vi "Local Variables.vi"() -> ()   [LabVIEW 2016]
panel:
  out "Stop":bool
  out "Boolean 3":bool
  out "Boolean 2":bool
  out "Boolean":bool
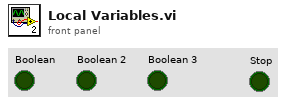
[diagram p1: front panel]
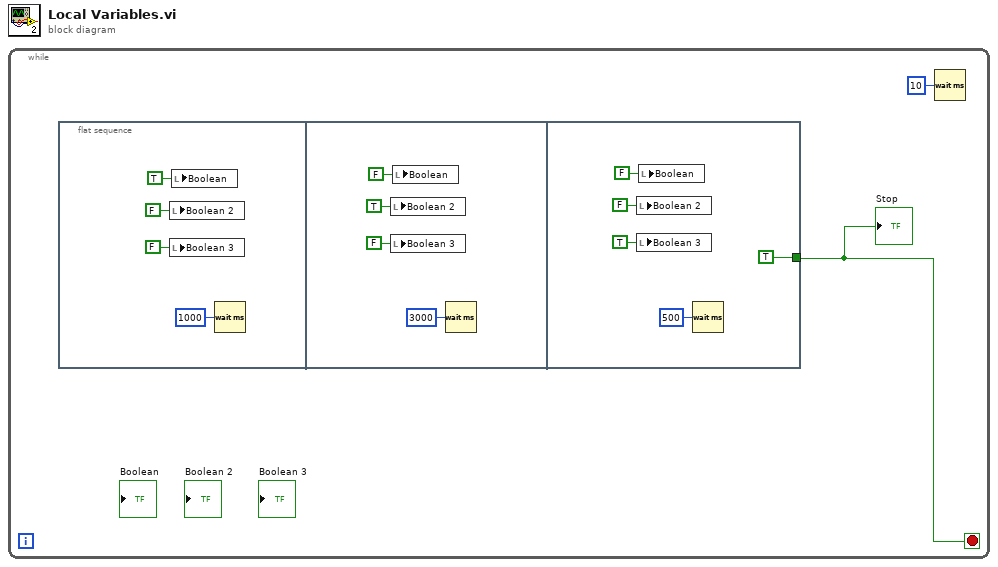
[diagram p0: block diagram]
diagram:
  n1 = while {
    stop <- w2 stop-if-true
    n2 = flat-sequence {
      tunnel: [TRUE] -> w2
      frame #0 {
        n3 = local write "Boolean 2"(FALSE ("Boolean 2")) -> ()
        n4 = local write "Boolean 3"(FALSE ("Boolean 3")) -> ()
        n5 = local write "Boolean"(TRUE ("Boolean")) -> ()
        n6 = Wait (ms)(milliseconds to wait=u32 1000) -> ()  [unwired: 1 out]
      }
      frame #1 {
        n7 = local write "Boolean 2"(TRUE ("Boolean 2")) -> ()
        n8 = local write "Boolean 3"(FALSE ("Boolean 3")) -> ()
        n9 = local write "Boolean"(FALSE ("Boolean")) -> ()
        n10 = Wait (ms)(milliseconds to wait=u32 3000) -> ()  [unwired: 1 out]
      }
      frame #2 {
        n11 = local write "Boolean 2"(FALSE ("Boolean 2")) -> ()
        n12 = local write "Boolean 3"(TRUE ("Boolean 3")) -> ()
        n13 = local write "Boolean"(FALSE ("Boolean")) -> ()
        n14 = Wait (ms)(milliseconds to wait=u32 500) -> ()  [unwired: 1 out]
      }
    }
    n15 = Wait (ms)(milliseconds to wait=u32 10) -> ()  [unwired: 1 out]
    "Stop" <- w2
  }
